vi "Propkonstant.vi"() -> ()   [LabVIEW 2024]
panel:
  in  "stop":bool
  out "Voltage V":dbl
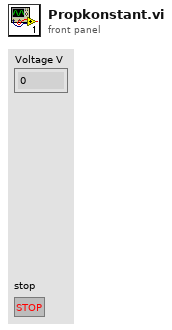
[diagram p1: front panel]
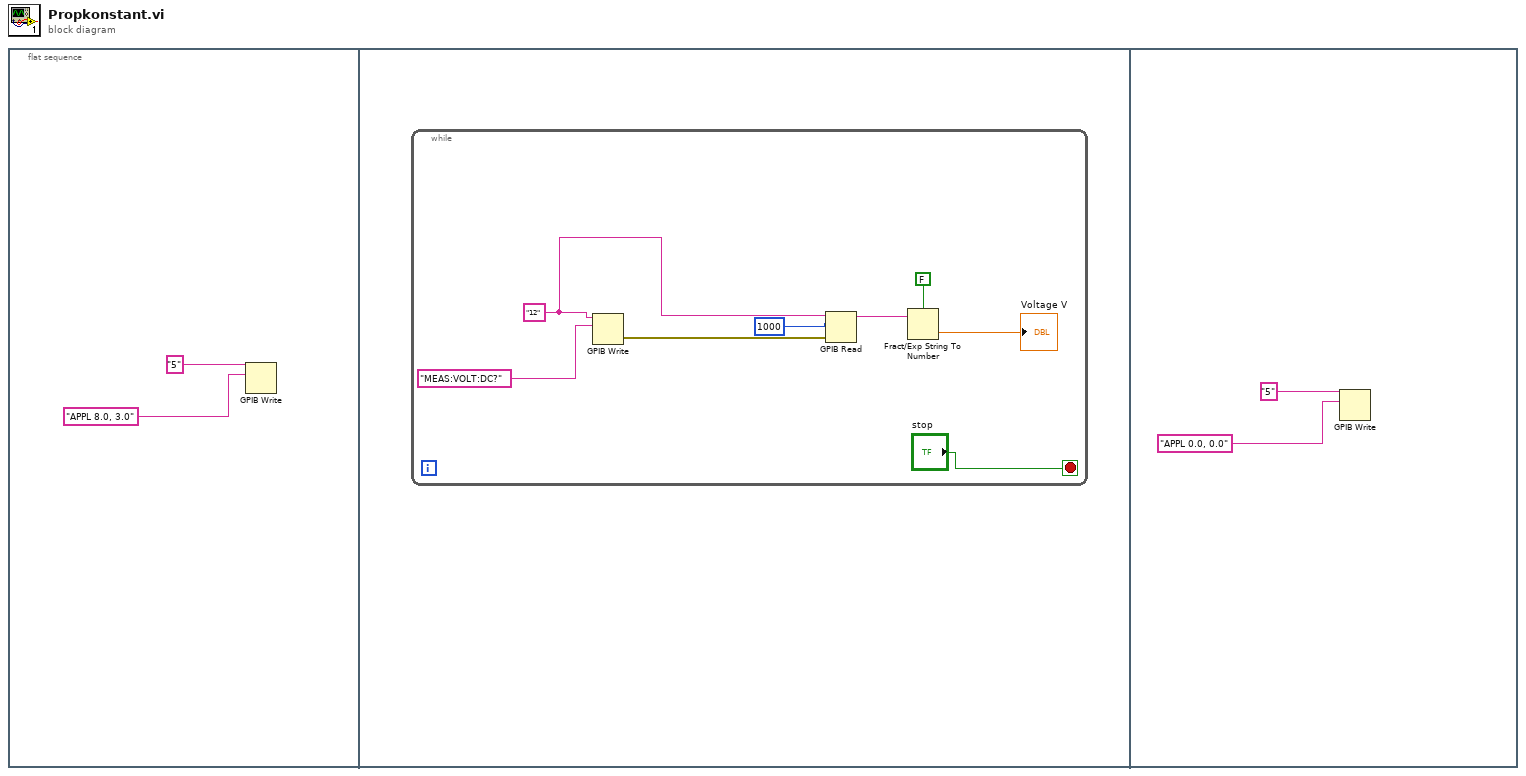
[diagram p0: block diagram]
diagram:
  n1 = flat-sequence {
    frame #0 {
      n2 = GPIB Write(0:"5" ("address string"), 1:"APPL 8.0, 3.0" ("data")) -> ()  [unwired: 3 in, 2 out]
    }
    frame #1 {
      n3 = while {
        stop <- "stop" stop-if-true
        w8 = "12" ("address string")
        n4 = GPIB Write(0:w8, 1:"MEAS:VOLT:DC?" ("data")) -> (6:w10:errorcluster)  [unwired: 3 in, 1 out]
        n5 = GPIB Read(0:w8, 1:1000 ("byte count"), 3:w10) -> (5:w6:string)  [unwired: 2 in, 2 out]
        n6 = Fract/Exp String To Number(use system decimal point (T)=FALSE, string=w6) -> (number=→"Voltage V":dbl)  [unwired: 2 in, 1 out]
      }
    }
    frame #2 {
      n7 = GPIB Write(0:"5" ("address string"), 1:"APPL 0.0, 0.0" ("data")) -> ()  [unwired: 3 in, 2 out]
    }
  }
